vi "Servo Set Pulse Width N Channels.vi"(8 "Error In":errorcluster, 9 "Pulse Widths (uS)":u16[](array[numeric]), 10 "Servo Channels":u8[](array[numeric]), 11 "LINX Resource":T1) -> (0 "Error Out":errorcluster, 3 "LINX Resource":T1)   [LabVIEW 2014, in "LMH-LINX.lvlib" / "Servo.lvlib"]
doc: "Set the pulse width of the specified servo channel.\n\nA pulse width of 1500uS is typically the center point of rotation (90 degrees). Most servos can rotate between 1000 and 2000 uS but the actual limits will vary depending on the specific servo.s"
uses:
  Servo.lvlib
  Private/Type Defs/LINX Ref.ctl
  Private/Type Defs/Platform.ctl
  Private/Type Defs/Interface.ctl
  Private/Device/Type Defs/LINX Device Config.ctl
  Private/Device/Type Defs/TCP Config.ctl
  Private/Device/Type Defs/Channels.ctl
  Private/Type Defs/Peripheral.ctl
  Private/Type Defs/Error Type.ctl
  LMH-LINX.lvlib
  Private/Device/Device.lvlib
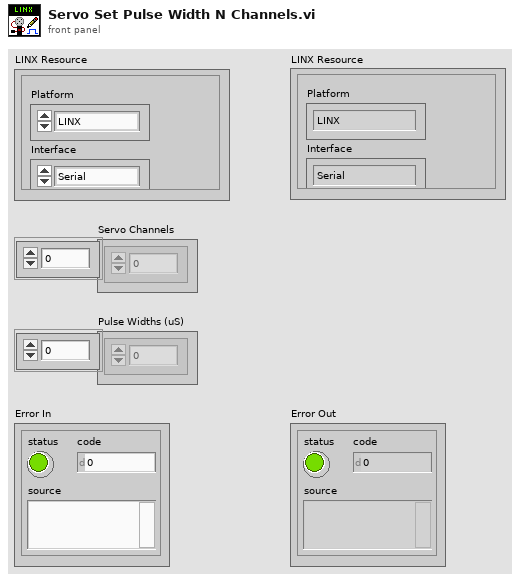
[diagram p1: front panel]
types:
  T1 = typedef "LMH-LINX.lvlib/LINX Ref.ctl" = cluster{"Platform":T2, "Interface":T3, "LINX Device Config":T4}
  T2 = typedef "LMH-LINX.lvlib/Platform.ctl" = enum16{"LINX", "myRIO"}
  T3 = typedef "LMH-LINX.lvlib/Interface.ctl" = enum16{"Serial", "TCP"}
  T4 = typedef "LMH-LINX.lvlib/Device.lvlib/LINX Device Config.ctl" = cluster{"Interface":T3, "COM Port":refnum<visa-resource-name>, "TCP Configuration":T5, "Device Family":u8, "Device ID":u8, "Device Name":string, "TCP Ref":refnum<k5>, "Channels":T6}
  T5 = typedef "LMH-LINX.lvlib/Device.lvlib/TCP Config.ctl" = cluster{"IP Address":string, "Port":u16}
  T6 = typedef "LMH-LINX.lvlib/Channels.ctl" = cluster{"DI":u8[], "DO":u8[], "AI":u8[], "AO":u8[], "PWM":u8[], "QE":u8[], "UART":u8[], "I2C 2":u8[], "SPI":u8[], "CAN":u8[], "Servo":u8[], "AI Ref (V)":dbl, "AO Ref (V)":dbl, "AO Resolution (Bits)":u8}
  T7 = typedef "LMH-LINX.lvlib/Peripheral.ctl" = enum8{"DI", "DO", "AI", "AO", "PWM", "QE", "UART", "I2C", "SPI", "CAN", "Servo"}
  T8 = typedef "LMH-LINX.lvlib/Error Type.ctl" = enum16{"Unknown", "Timeout", "Corrupt Return Packet", "Unable To Connect", "Command Not Supported", "Channel DNE", "Invalid COM Config", "Firmware Version Mismatch", "myRIO Support", "CMD Specific Error"}
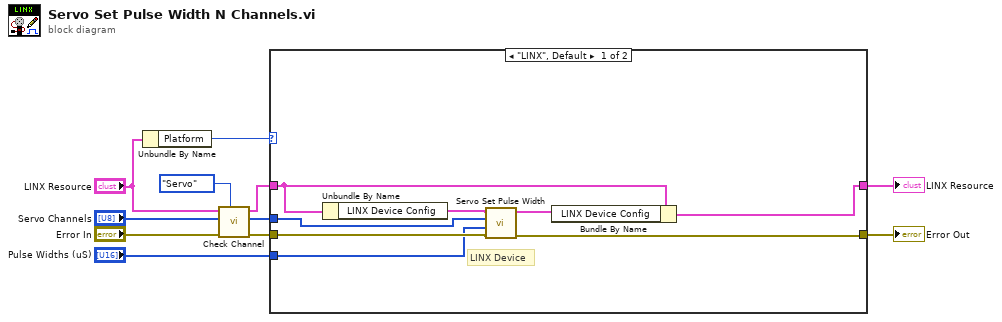
[diagram p0: block diagram]
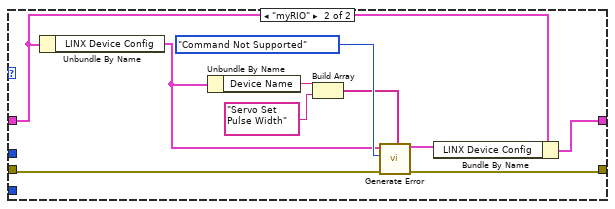
[diagram p2: hidden frame]
diagram:
  n1 = Unbundle By Name("LINX Resource") -> ("Platform"=w11:T2)
  n2 = call "Check Channel.vi"("Peripheral"=Peripheral."Servo", "Error In"="Error In", "Channels"="Servo Channels", "LINX Resource"="LINX Resource") -> ("Error Out"=w8:errorcluster, "Channels"=w7:u8[], "LINX Resource"=w5:T1)  [unwired: 5 in]
  n3 = case shown="\"LINX\", Default" w11 {
    tunnel: w8 -> [w15 w29]
    tunnel: w5 -> [w19 w22]
    tunnel: [w14 w28] -> w10
    tunnel: [w18 w20] -> w9
    tunnel: w7 -> [w13 _]
    tunnel: "Pulse Widths (uS)" -> [w12 _]
    frame "LINX", Default {
      # "LINX Device"
      n4 = Unbundle By Name(w19) -> ("LINX Device Config"=w17:T4)
      n5 = call "Servo Set Pulse Width.vi"("Error In"=w15, "Pulse Widths (uS)"=w12, "Channels"=w13, "LINX Device Config"=w17) -> ("Error Out"=w14:errorcluster, "LINX Device Config"=w16:T4)  [unwired: 6 in]
      n6 = Bundle By Name(cluster=w19, "LINX Device Config"=w16) -> (w18:T1)
    }
    frame "myRIO" {
      n7 = Unbundle By Name(w22) -> ("LINX Device Config"=w23:T4)
      n8 = Unbundle By Name(w23) -> ("Device Name"=w27:string)
      n9 = Build Array(w27, "Servo Set Pulse Width") -> (w24:string[])
      n10 = call "Generate Error.vi"("Error In"=w29, "Arguments"=w24, "Error Type"=Error_Type."Command Not Supported", "LINX Device Config"=w23) -> ("Error Out"=w28:errorcluster, "LINX Device Config"=w21:T4)  [unwired: 6 in]
      n11 = Bundle By Name(cluster=w22, "LINX Device Config"=w21) -> (w20:T1)
    }
  }
  "Error Out" <- w10
  "LINX Resource" <- w9
